vi "Forebrain 2.vi"() -> ()   [LabVIEW 2011]
uses:
  MDF.ctl
  Behaviour.ctl
  Position.ctl
  WhereAmI.ctl
  ForebrainCmd.ctl
panel:
  out "Forebrain Command":T1
  out "Current State 2":i32
  out "Draw?":bool
  in  "stop":bool
  in  "Tab Control":enum32{"Mission Planning", "Auto-Mode"}(tab)
  in  "Behaviour":T2
  out "No. of Waypoints":i16
  out "Waypoint Index":i16
  in  "Speed":dbl(slide) scale=0.0..10.0
  out "Mission Definition":picture
  in  "path to PNG file":path
  out "MDF":T3[](array[typedef])
  out "Buoy2":T4
  out "Buoy1":T4
  out "Dock":T4
  out "Real-Time MDF":T3[](array[typedef])
  out "Boat":T5
  out "ActCmd":dbl[](array[numeric])
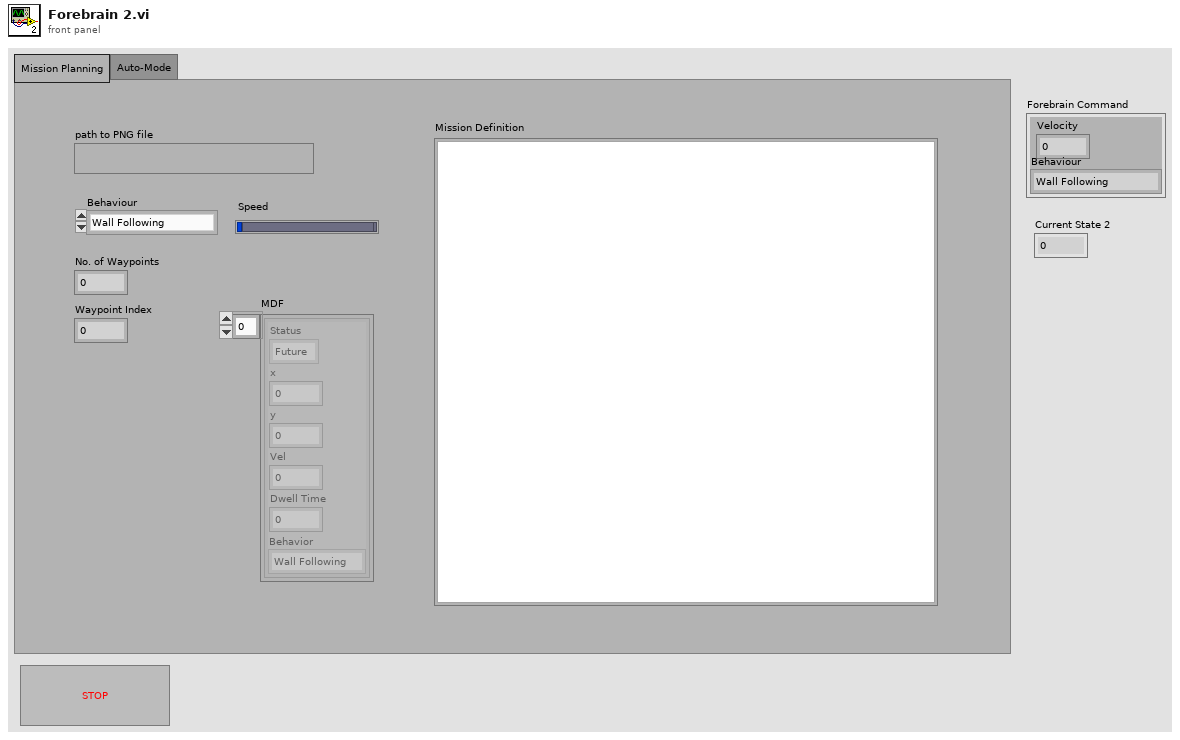
[diagram p1: front panel]
types:
  T1 = typedef "ForebrainCmd.ctl" = cluster{"Velocity":dbl, "Behaviour":T2}
  T2 = typedef "Behaviour.ctl" = enum16{"Wall Following", "Open Transit", "Find Barge", "Push Barge", "Go Home"}
  T3 = typedef "MDF.ctl" = cluster{"Status":enum16{"Past", "Current", "Future"}, "x":dbl, "y":dbl, "Vel":dbl, "Dwell Time":dbl, "Behavior":T2}
  T4 = typedef "Position.ctl" = cluster{"X":sgl, "Y":sgl}
  T5 = typedef "WhereAmI.ctl" = cluster{"x":sgl, "y":sgl, "Boat\nHeading":sgl}
  T6 = cluster{"Status":enum16{"Past", "Current", "Future"}, "x":dbl, "y":dbl, "Vel":dbl, "Dwell Time":dbl, "Behavior":T2}[]
  T7 = typedef "imagedata.ctl" = cluster{"image type":i32, "image depth":i32, "image":u8[], "mask":u8[], "colors":u32[], "Rectangle":cluster{"left":i16, "top":i16, "right":i16, "bottom":i16}}
  T8 = cluster{"Status":enum16{"Past", "Current", "Future"}, "x":dbl, "y":dbl, "Vel":dbl, "Dwell Time":dbl, "Behaviour":T2}
  T9 = cluster{"Width":u16, "Style":enum32{"Solid", "Dash", "Dot", "DashDot", "DashDotDot"}}
  T10 = typedef "LVMouseTypeDef.ctl" = cluster{"Mouse Position":cluster{"X":i32, "Y":i32}, "Mouse Modifiers":cluster{"Button Down":bool, "Shift Mod":bool, "Menu Mod":bool, "Option Mod":bool}}
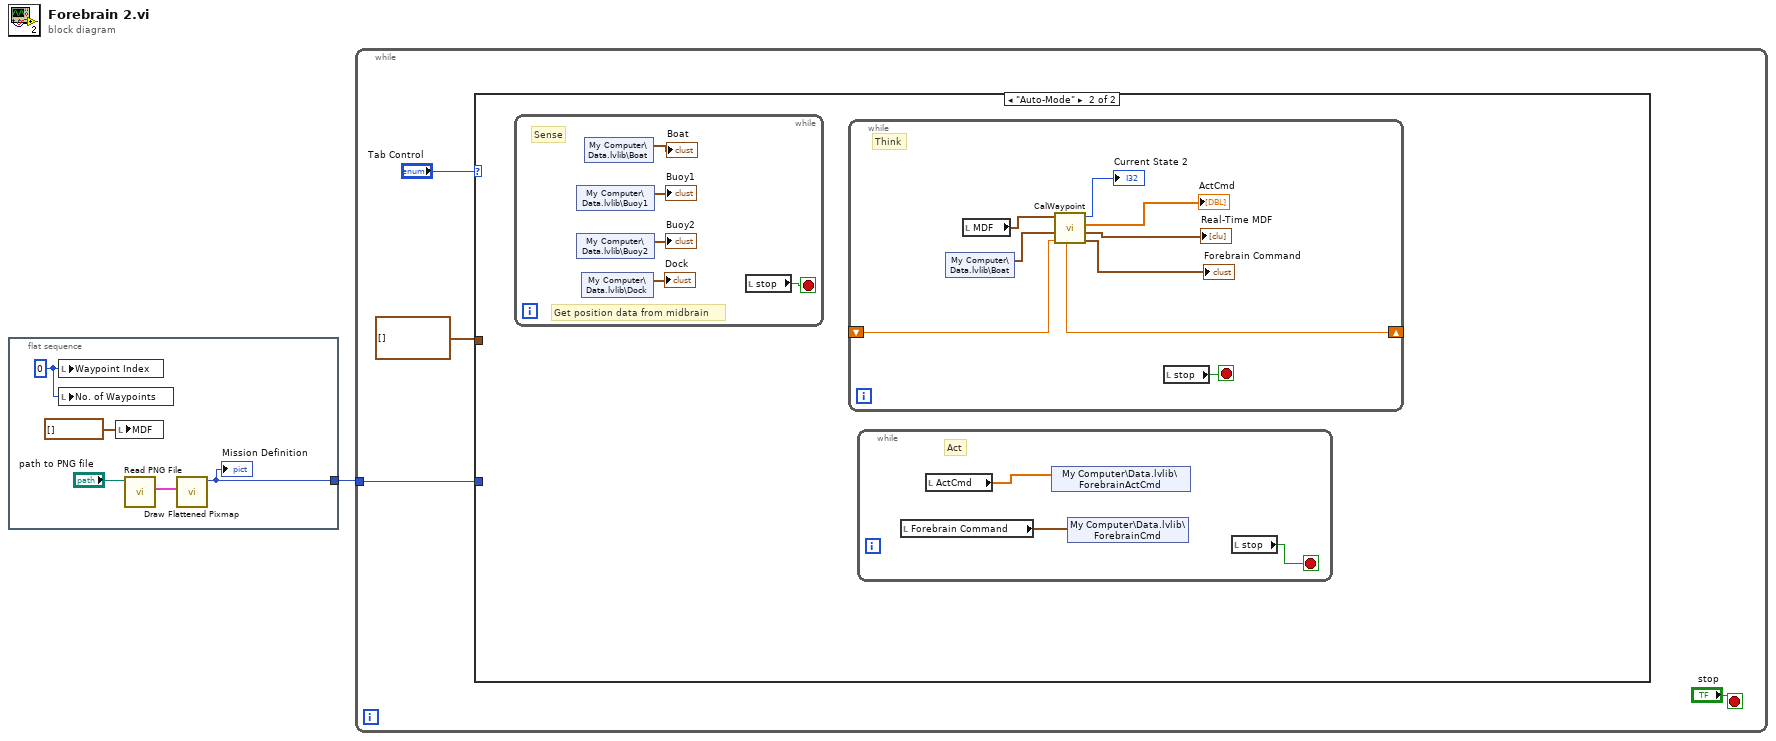
[diagram p0: block diagram]
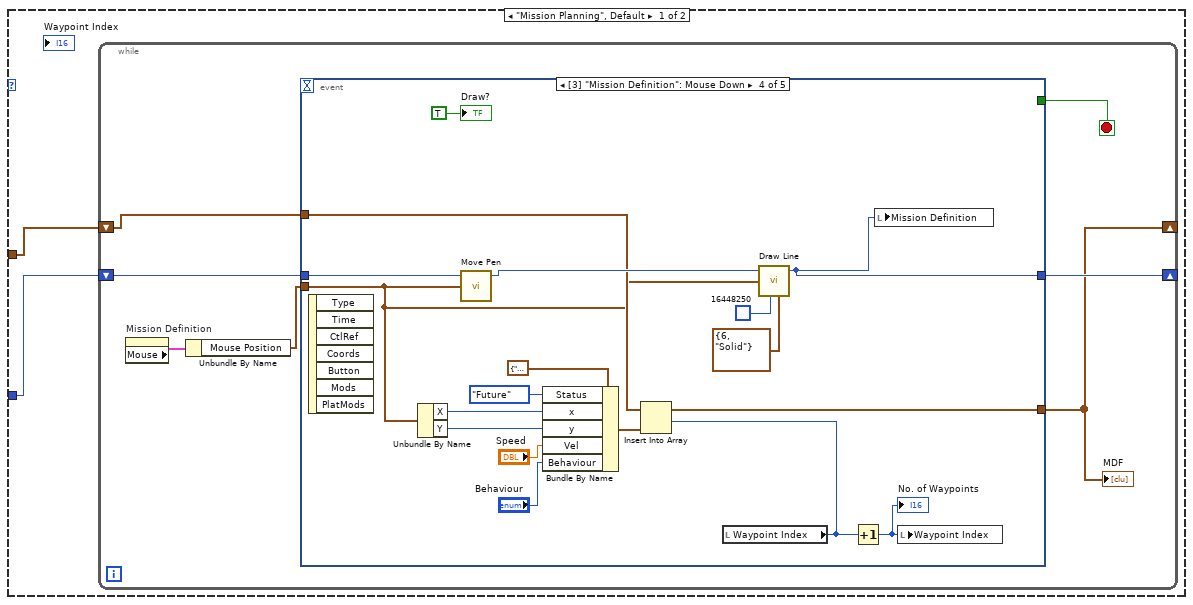
[diagram p2: hidden frame]
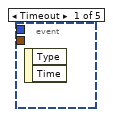
[diagram p3: hidden frame]
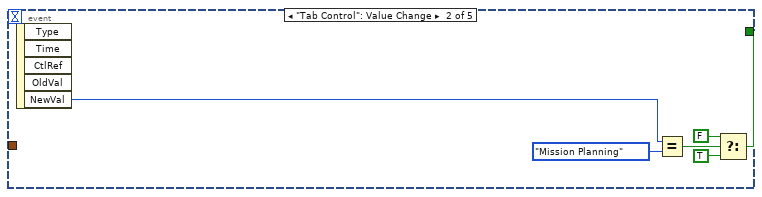
[diagram p4: hidden frame]
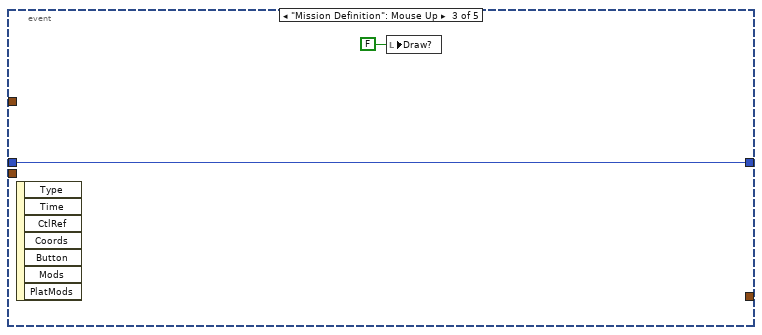
[diagram p5: hidden frame]
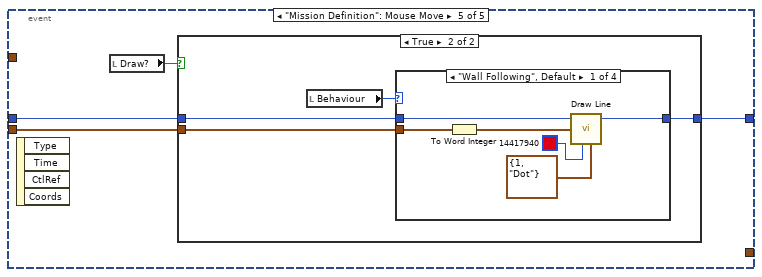
[diagram p6: hidden frame]
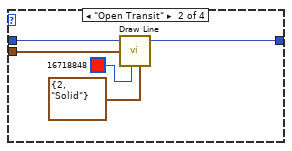
[diagram p8: hidden frame]
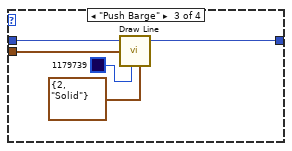
[diagram p9: hidden frame]
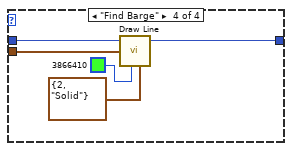
[diagram p10: hidden frame]
diagram:
  n1 = flat-sequence {
    tunnel: [w4] -> w1
    frame #0 {
      w3 = i16 0 ("No. of Waypoints")
      n2 = local write "Waypoint Index"(w3) -> ()
      n3 = local write "No. of Waypoints"(w3) -> ()
      n4 = local write "MDF"(T6 [] ("MDF")) -> ()
      n5 = call <vilib>:"Read PNG File.vi"("path to PNG file"="path to PNG file") -> ("image data"=w6:T7)  [unwired: 8 in, 2 out]
      n6 = call <vilib>:"Draw Flattened Pixmap.vi"("image data"=w6) -> ("new picture"=w4:picture)  [unwired: 8 in]
      "Mission Definition" <- w4
    }
  }
  n7 = while {
    tunnel: w1 -> [w8]
    stop <- "stop" stop-if-true
    n8 = case shown="\"Auto-Mode\"" "Tab Control" {
      tunnel: w8 -> [w12 _]
      tunnel: T3[] [] ("MDF") -> [w11 _]
      frame "Mission Planning", Default {
        n9 = while {
          shift-right: [w15] -> _
          shift-left: w11 -> [w19]
          shift-right: [w16] -> _
          shift-left: w12 -> [w17]
          stop <- w18 stop-if-true
          n10 = property on="Mission Definition" class="Pict"() -> ("Mouse"=w14:T10)  [unwired: 2 in, 2 out]
          n11 = Unbundle By Name(w14) -> ("Mouse Position"=w13:cluster{"X":i32, "Y":i32})
          n12 = event shown="[3] \"Mission Definition\": Mouse Down" {
            selector: _ -> [_ _ _ _ _]
            dyn-events: _ -> [_ _ _ _ _]
            timeout: _ -> [_ _ _ _ _]
            tunnel: w19 -> [_ _ _ w42 _]
            tunnel: [_ _ _ w35 _] -> w15
            tunnel: [_ w20 _ _ _] -> w18
            tunnel: w17 -> [_ _ w26 w34 w47]
            tunnel: [_ _ w26 w28 w46] -> w16
            tunnel: w13 -> [_ _ _ w29 w48]
            event Timeout {
              n13 = event-data() -> ()  [unwired: 1 in, 2 out]
            }
            event "Tab Control": Value Change {
              n14 = event-data() -> ("NewVal"=w25:enum32{"Mission Planning", "Auto-Mode"})  [unwired: 1 in, 4 out]
              n15 = Equal?(x=w25, y=enum32{"Mission Planning", "Auto-Mode"}."Mission Planning") -> (x = y?=w23:bool)
              n16 = Select(t=FALSE, s=w23, f=TRUE) -> (s? t:f=w20:bool)
            }
            event "Mission Definition": Mouse Up {
              n17 = event-data() -> ()  [unwired: 1 in, 7 out]
              n18 = local write "Draw?"(FALSE ("Draw?")) -> ()
            }
            event "Mission Definition": Mouse Down {
              n19 = event-data() -> ()  [unwired: 1 in, 7 out]
              n20 = Unbundle By Name(w29) -> ("X"=w41:i32, "Y"=w40:i32)
              n21 = call <vilib>:"Move Pen.vi"("new position"=w29, "picture"=w34) -> ("new picture"=w45:picture)  [unwired: 3 in]
              n22 = Bundle By Name(cluster=T8 {"Status"=enum."Future", "x"=0.0, "y"=0.0, "Vel"=0.0, "Dwell Time"=0.0, "Behaviour"=enum."Wall Following"} ("MissionDefinitionFile"), "Status"=enum16{"Past", "Current", "Future"}."Future", "x"=w41, "y"=w40, "Vel"="Speed", "Behaviour"="Behaviour") -> (w31:T8)
              n23 = local read "Waypoint Index"() -> (w39:i16)
              n24 = Insert Into Array(array=w42, index=w39, new element=w31) -> (w35:T3[])
              n25 = call <vilib>:"Draw Line.vi"("picture"=w45, "end point"=w29, "color(black)"=u32 16448250, "pen"=T9 {"Width"=6, "Style"=enum."Solid"}) -> ("new picture"=w28:picture)  [unwired: 5 in]
              n26 = Increment(x=w39) -> (x+1=w38:i16)
              "No. of Waypoints" <- w38
              n27 = local write "Mission Definition"(w28) -> ()
              n28 = local write "Waypoint Index"(w38) -> ()
              "Draw?" <- TRUE ("Draw?")
            }
            event "Mission Definition": Mouse Move {
              n29 = event-data() -> ()  [unwired: 1 in, 4 out]
              n30 = local read "Draw?"() -> (w49:bool)
              n31 = case shown="True" w49 {
                tunnel: w48 -> [_ w54]
                tunnel: w47 -> [w50 w53]
                tunnel: [w50 w52] -> w46
                frame False {
                }
                frame True {
                  n32 = local read "Behaviour"() -> (w51:T2)
                  n33 = case shown="\"Wall Following\", Default" w51 {
                    tunnel: w54 -> [w56 w65 w70 w75]
                    tunnel: w53 -> [w60 w62 w67 w72]
                    tunnel: [w57 w61 w66 w71] -> w52
                    frame "Wall Following", Default {
                      n34 = To Word Integer(number=w56) -> (16bit integer=w55:cluster{"X":i16, "Y":i16})
                      n35 = call <vilib>:"Draw Line.vi"("picture"=w60, "end point"=w55, "color(black)"=u32 14417940, "pen"=T9 {"Width"=1, "Style"=enum."Dot"}) -> ("new picture"=w57:picture)  [unwired: 5 in]
                    }
                    frame "Open Transit" {
                      n36 = call <vilib>:"Draw Line.vi"("picture"=w62, "end point"=w65, "color(black)"=u32 16718848, "pen"=T9 {"Width"=2, "Style"=enum."Solid"}) -> ("new picture"=w61:picture)  [unwired: 5 in]
                    }
                    frame "Push Barge" {
                      n37 = call <vilib>:"Draw Line.vi"("picture"=w67, "end point"=w70, "color(black)"=u32 1179739, "pen"=T9 {"Width"=2, "Style"=enum."Solid"}) -> ("new picture"=w66:picture)  [unwired: 5 in]
                    }
                    frame "Find Barge" {
                      n38 = call <vilib>:"Draw Line.vi"("picture"=w72, "end point"=w75, "color(black)"=u32 3866410, "pen"=T9 {"Width"=2, "Style"=enum."Solid"}) -> ("new picture"=w71:picture)  [unwired: 5 in]
                    }
                  }
                }
              }
            }
          }
          "MDF" <- w15
        }
      }
      frame "Auto-Mode" {
        n39 = while {
          stop <- w89 stop-if-true
          # "Get position data from midbrain"
          # "Sense"
          n40 = shared-variable "My Computer\\Data.lvlib\\Buoy1"() -> (→"Buoy1":T4)  [unwired: 1 in, 1 out]
          n41 = shared-variable "My Computer\\Data.lvlib\\Buoy2"() -> (→"Buoy2":T4)  [unwired: 1 in, 1 out]
          n42 = shared-variable "My Computer\\Data.lvlib\\Dock"() -> (→"Dock":T4)  [unwired: 1 in, 1 out]
          n43 = shared-variable "My Computer\\Data.lvlib\\Boat"() -> (→"Boat":T5)  [unwired: 1 in, 1 out]
          n44 = local read "stop"() -> (w89:bool)
        }
        n45 = while {
          shift-right: [w82] -> _
          shift-left: _ -> [w81]
          stop <- w87 stop-if-true
          # "Think"
          n46 = shared-variable "My Computer\\Data.lvlib\\Boat"() -> (w83:T5)  [unwired: 1 in, 1 out]
          n47 = local read "MDF"() -> (w86:T3[])
          n48 = call "CalWaypoint.vi"("CurrentSteerAngle"=w81, "WhereAmI?"=w83, "MDD In"=w86) -> ("Forebrain Command"=→"Forebrain Command":T1, "MDF Out"=→"Real-Time MDF":T3[], "ActCommand"=→"ActCmd":dbl[], "Current State"=→"Current State 2":i32, "SteerAngle"=w82:dbl)  [unwired: 2 in, 2 out]
          n49 = local read "stop"() -> (w87:bool)
        }
        n50 = while {
          stop <- w78 stop-if-true
          # "Act"
          n51 = local read "Forebrain Command"() -> (w76:T1)
          n52 = local read "ActCmd"() -> (w77:dbl[])
          n53 = shared-variable "My Computer\\Data.lvlib\\ForebrainActCmd"(w77) -> ()  [unwired: 1 in, 1 out]
          n54 = shared-variable "My Computer\\Data.lvlib\\ForebrainCmd"(w76) -> ()  [unwired: 1 in, 1 out]
          n55 = local read "stop"() -> (w78:bool)
        }
      }
    }
  }
